vi "Set Item Property (Dependent Node Pointer).vi"(8 "error in (no error)":errorcluster, 9 "Dependent Node Ref":T1=18446744073709551615 format="%.0x", 10 "Property Name":string, 11 "Item Ref in":T1 format="%.0x") -> (0 "error out":errorcluster, 3 "Item Ref out":T1 format="%.0x", 4 "Replaced":bool)   [LabVIEW 2026, in "Custom Devices Storage.lvlib"]
uses:
  Custom Devices Storage.lvlib
  <vilib>/NI VeriStand/Custom Device API/Custom Device Item Ref.ctl
  C:/Users/Administrator/Desktop/Jatin/All DNC DLLs/NationalInstruments.VeriStand.SystemDefinitionAPI.dll
  Jatin/All DNC DLLs/NationalInstruments.VeriStand.SystemDefinitionAPI.dll
  <vilib>/NI VeriStand/Custom Device API/Custom Device API.lvlib
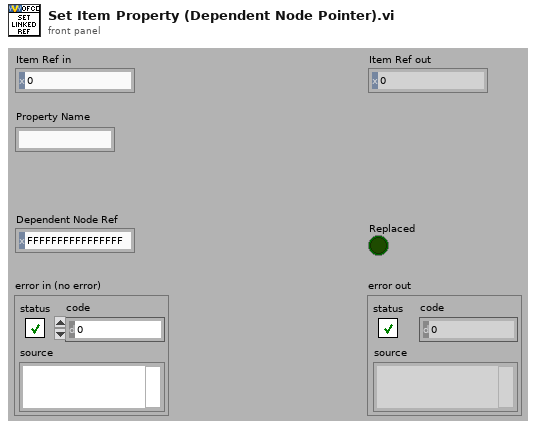
[diagram p1: front panel]
types:
  T1 = typedef "Custom Device API.lvlib/Custom Device Item Ref.ctl" = u64
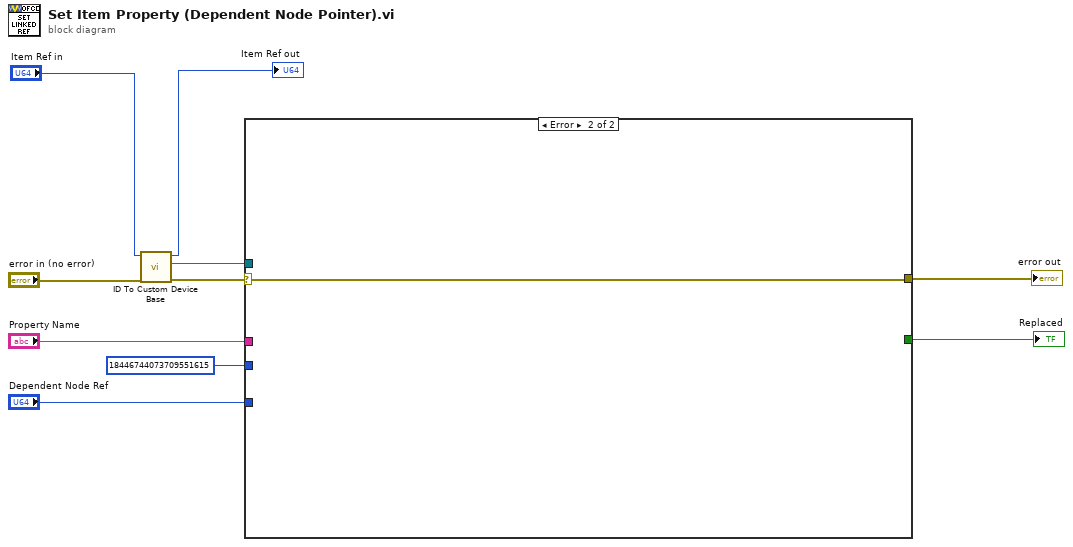
[diagram p0: block diagram]
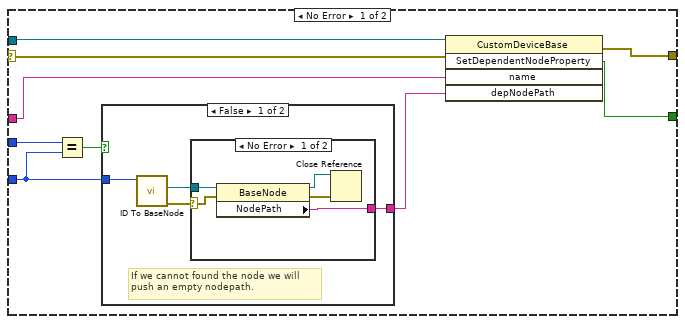
[diagram p2: hidden frame]
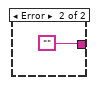
[diagram p3: hidden frame]
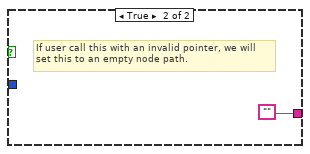
[diagram p4: hidden frame]
diagram:
  n1 = call "ID To Custom Device Base.vi"("error in (no error)"="error in (no error)", "ID in"="Item Ref in") -> ("error out"=w7:errorcluster, "NationalInstruments.VeriStand.SystemDefinitionAPI.CustomDeviceBase"=w6:refnum<k39>, "ID out"=→"Item Ref out":u64)  [unwired: 7 in]
  n2 = case shown="Error" w7 {
    selector: w7 -> [w15 w31]
    tunnel: w6 -> [w19 _]
    tunnel: "Property Name" -> [w18 _]
    tunnel: "Dependent Node Ref" -> [w11 _]
    tunnel: [w17 w31] -> w3
    tunnel: [w16 _] -> w2
    tunnel: T1 18446744073709551615 ("Dependent Node Ref") -> [w13 _]
    frame No Error {
      n3 = Equal?(x=w13, y=w11) -> (x = y?=w12:bool)
      n4 = case shown="False" w12 {
        tunnel: [w21 ""] -> w14
        tunnel: w11 -> [w20 _]
        frame False {
          # "If we cannot found the node we will\npush an empty nodepath."
          n5 = call "ID To BaseNode.vi"("ID in"=w20) -> ("error out"=w23:errorcluster, "NationalInstruments.VeriStand.SystemDefinitionAPI.BaseNode"=w22:refnum<k39>)  [unwired: 8 in, 1 out]
          n6 = case shown="No Error" w23 {
            selector: w23 -> [w24 _]
            tunnel: w22 -> [w28 _]
            tunnel: [w27 ""] -> w21
            frame No Error {
              n7 = property class="BaseNode"(reference=w28, error in=w24) -> (reference out=w25:refnum<k39>, error out=w26:errorcluster, "NodePath"=w27:string)
              n8 = Close Reference(reference=w25, error in (no error)=w26) -> ()  [unwired: 1 out]
            }
            frame Error {
            }
          }
        }
        frame True {
          # "If user call this with an invalid pointer, we will\nset this to an empty node path."
        }
      }
      n9 = invoke class="CustomDeviceBase" method="SetDependentNodeProperty"(reference=w19, error in=w15, "name"=w18, "depNodePath"=w14) -> (error out=w17:errorcluster, "SetDependentNodeProperty"=w16:bool)  [unwired: 1 in, 3 out]
    }
    frame Error {
    }
  }
  "error out" <- w3
  "Replaced" <- w2
